vi "Destroy IntelliSense Control.vi"(0 "IntelliSense Control":refnum<class "IntelliSenseStringControl.lvclass">, 11 "error in":errorcluster) -> (4 "Str Ctl Refnum":refnum<vi>, 15 "error out":errorcluster)   [LabVIEW 2016, in "StringIntelliSense.lvlib" / "IntelliSenseStringControl.lvclass"]
uses:
  IntelliSenseStringControl.lvclass
  IntelliSenseStringControl.lvclass/IntelliSenseStringControl.ctl
  Suggestions IO/base/SuggestionIObase.lvclass
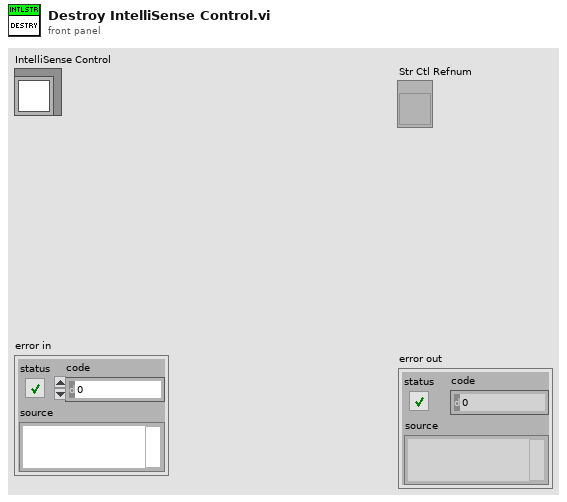
[diagram p1: front panel]
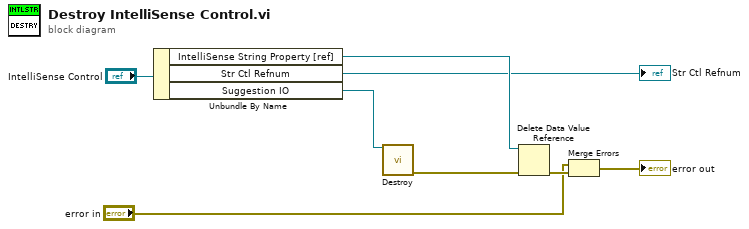
[diagram p0: block diagram]
diagram:
  n1 = Unbundle By Name("IntelliSense Control") -> ("IntelliSense String Property [ref]"=w5:refnum<data-value>, "Str Ctl Refnum"=→"Str Ctl Refnum":refnum<vi>, "Suggestion IO"=w7:refnum<class "SuggestionIObase.lvclass">)
  n2 = call-dynamic "Destroy.vi"("Suggestion IO in"=w7) -> ("error out"=w6:errorcluster)  [unwired: 13 in, 1 out]
  n3 = Delete Data Value Reference(data value reference=w5, error in=w6) -> (error out=w4:errorcluster)  [unwired: 1 out]
  n4 = Merge Errors("error in", w4) -> (→"error out":errorcluster)
